vi "Main.vi"() -> ()   [LabVIEW 2014]
uses:
  MAVLink_example.llb/Heartbeat.ctl
  MAVLink_example.llb/Battery Info.ctl
  MAVLink_example.llb/Raw IMU.ctl
  MAVLink_example.llb/Position.ctl
  MAVLink_example.llb/Attitude.ctl
  <vilib>/myRIO/Common/Instrument Driver Framework/myRIO v1.0/PWM/vis/myRIO v1.1 Open PWM.vi
  <vilib>/myRIO/Common/Instrument Driver Framework/myRIO v1.0/UART/vis/myRIO v1.0 Close UART.vi
  <vilib>/myRIO/Common/Instrument Driver Framework/Utilities/vis/Validate Channels.vi
  <vilib>/myRIO/Common/Instrument Driver Framework/myRIO v1.0/PWM/vis/myRIO v1.0 Reserve PWM.vi
  <vilib>/myRIO/Common/Instrument Driver Framework/myRIO v1.0/PWM/vis/myRIO v1.0 Build MUX Configuration PWM.vi
  <vilib>/myRIO/Common/Instrument Driver Framework/myRIO v1.0/Resource Manager/vis/myRIO v1.0 Reserve Channel List.vi
  <vilib>/myRIO/Common/Instrument Driver Framework/myRIO v1.0/Resource Manager/vis/myRIO v1.0 Create Configuration List.vi
  <vilib>/myRIO/Common/Instrument Driver Framework/myRIO v1.0/Resource Manager/vis/myRIO v1.0 Reserve Channel.vi
  <vilib>/myRIO/Common/Instrument Driver Framework/myRIO v1.0/Resource Manager/vis/myRIO v1.0 Unreserve Channel.vi
  <vilib>/myRIO/Common/Instrument Driver Framework/myRIO v1.0/Resource Manager/vis/myRIO v1.0 Build Mutex Name.vi
  <vilib>/Utility/VariantDataType/GetNumericInfo.vi
  <vilib>/Utility/error.llb/Error Cluster From Error Code.vi
  <vilib>/myRIO/Common/Instrument Driver Framework/myRIO v1.0/myRIO v1.1 Open.vi
  <vilib>/myRIO/Common/Instrument Driver Framework/Utilities/vis/IO Manager.vi
  <vilib>/myRIO/Common/Instrument Driver Framework/Utilities/vis/Configuration Manager.vi
  <vilib>/myRIO/Common/Instrument Driver Framework/myRIO v1.0/Resource Manager/vis/myRIO v1.0 Configure IO.vi
  <vilib>/myRIO/Common/Instrument Driver Framework/myRIO v1.0/myRIO v1.0 Close.vi
  Web/Globals/globalAntena.vi
  <vilib>/myRIO/Common/Instrument Driver Framework/myRIO v1.0/PWM/vis/myRIO v1.0 Write PWM.vi
  MAVLink_example.llb/Global Vars.vi
  <vilib>/myRIO/Common/Instrument Driver Framework/Utilities/vis/FPGA Ref Manager.vi
  <vilib>/myRIO/Common/Instrument Driver Framework/myRIO v1.0/myRIO v1.0 Reset FPGA.vi
  <vilib>/myRIO/Common/Instrument Driver Framework/myRIO v1.0/IRQ/vis/myRIO v1.0 IRQ Info FGV.vi
  <vilib>/myRIO/Common/Instrument Driver Framework/myRIO v1.0/IRQ/vis/myRIO v1.0 Timer IRQ Info FGV.vi
  <vilib>/myRIO/Common/Instrument Driver Framework/myRIO v1.0/IRQ/vis/myRIO v1.0 ISR Agent.vi
  Web/Globals/globalAvion.vi
  <vilib>/myRIO/Instrument Drivers/Utilities/Utilities.lvlib
  <vilib>/myRIO/Instrument Drivers/Onboard IO/PWM/PWM.lvlib
panel:
  out "error out 2":errorcluster
  out "Attitude":T1
  out "Position":T2 {"Heading" format="%.2f"}
  out "Raw IMU":T3
  out "Battery Info":T4 {"Batt Voltage (V)" format="%.2f"; "Batt Current (Ah)" format="%.2f"}
  out "HeartBeat":T5 {"custom_mode" format="%x"}
  out "GPS Lock":bool
  out "Received Messages":u8[](array[numeric])
  out "# of HB":u32
  in  "stop":bool
  out "error out":errorcluster
  in  "Actualizar":bool
  out "Altitud Global":dbl
  out "Longitud Global":dbl
  out "Latitud Global":dbl
  in  "Altitud":dbl
  in  "Longitud":dbl
  in  "Latitud":dbl
  in  "Arriba":bool
  in  "Derecha":bool
  out "Duty Cycle  [E]":dbl(graph)
  out "Grados [E]":dbl(graph)
  out "offset [%FS] [E]":dbl
  out "duty cycle [%]  [E]":dbl
  out "pulse width [ms]  [E]":dbl=1.5
  in  "null offset 3":bool
  in  "freq [Hz] Elevación":dbl=50.0
  in  "Parar elevacion":bool
  in  "Kp elevación":dbl=0.05
  in  "Kp rotación":dbl=0.02
  out "Objeto detectado":bool
  in  "Parar rotacion":bool
  out "Grados  [R]":dbl(graph)
  out "Duty Cycle  [R]":dbl(graph)
  out "offset [%FS]  [R]":dbl
  in  "null offset 2":bool
  out "duty cycle [%]  [R]":dbl
  out "pulse width [ms]  [R]":dbl=1.5
  in  "freq [Hz] Rotación":dbl=50.0
  in  "milliseconds to wait":u32=200
  out "Frame Rate":dbl
  in  "Number of Erosion (Adv. Morphology 1)":i32=5
  out "Imagen procesada":T6(plugin-control)
  out "Centroid (Centroid 1)":cluster{"X Centroid":sgl, "Y Centroid":sgl} {"Y Centroid" format="%.2f"; "X Centroid" format="%.2f"}
  out "Number of Particles (Particle Analysis 1)":i32
  in  "Range (Threshold 1)":cluster{"Lower value":sgl, "Upper value":sgl}={"Lower value"=203.0, "Upper value"=255.0}
  in  "Stop (F)":bool
  # "PROCESADO IMAGEN"
  # "DIRECCION RASTREO ->"
  # "ROTACIÓN"
  # "ELEVACIÓN"
  # "POSICION ANTENA"
  # "GPS"
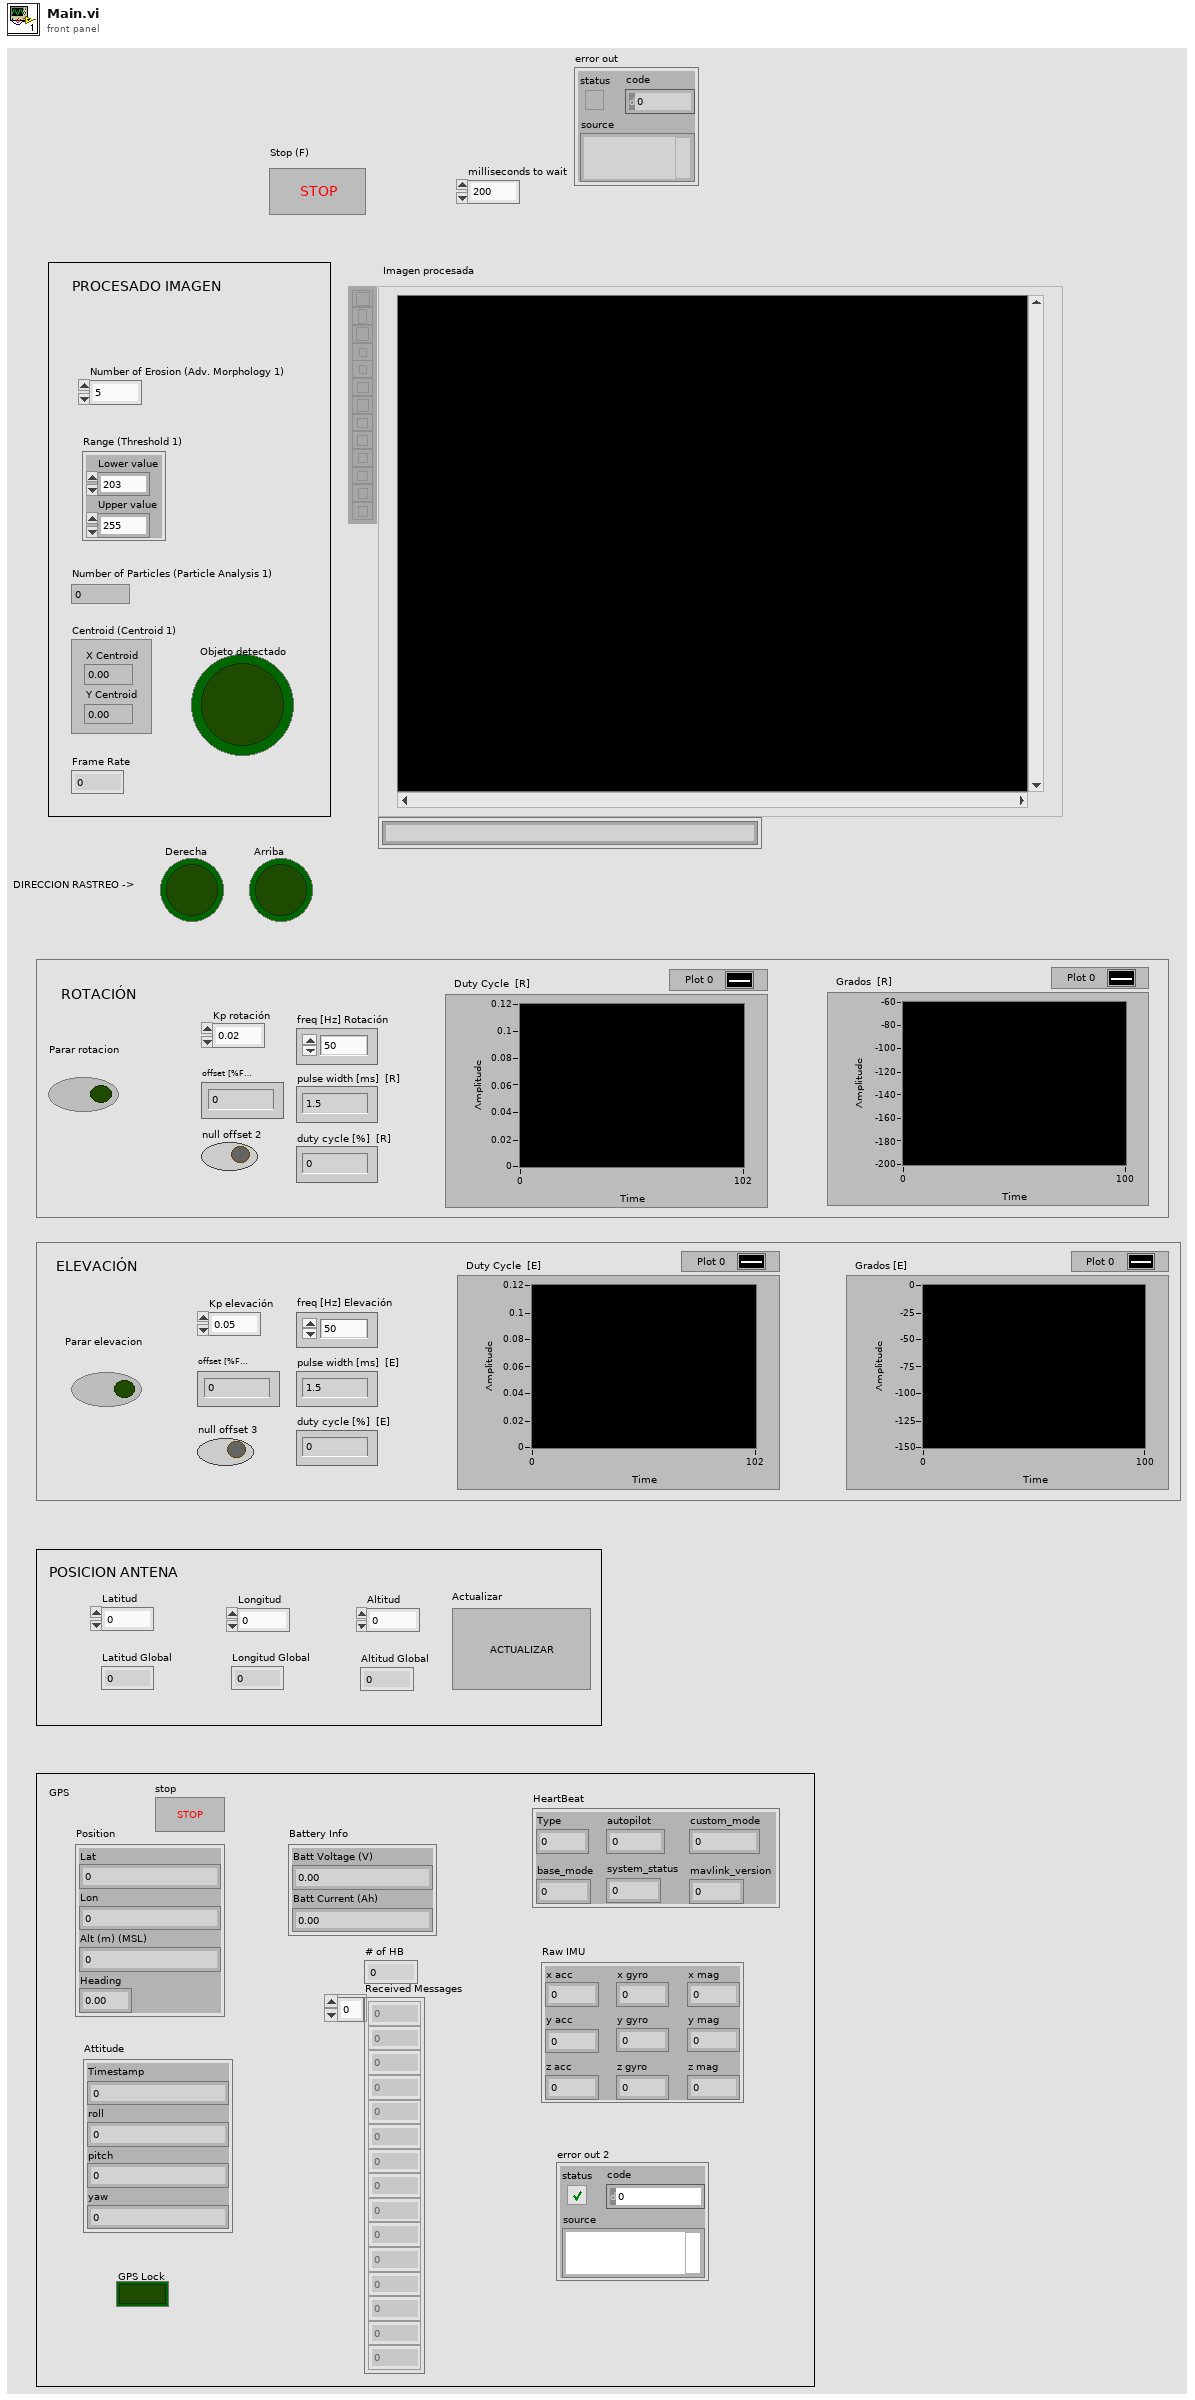
[diagram p1: front panel]
types:
  T1 = typedef "Attitude.ctl" = cluster{"Timestamp":u32, "roll":sgl, "pitch":sgl, "yaw":sgl}
  T2 = typedef "Position.ctl" = cluster{"Lat":sgl, "Lon":sgl, "Alt (m) (MSL)":sgl, "Heading":dbl}
  T3 = typedef "Raw IMU.ctl" = cluster{"x acc":i16, "y acc":i16, "z acc":i16, "x gyro":i16, "y gyro":i16, "z gyro":i16, "x mag":i16, "y mag":i16, "z mag":i16}
  T4 = typedef "Battery Info.ctl" = cluster{"Batt Voltage (V)":dbl, "Batt Current (Ah)":dbl}
  T5 = typedef "Heartbeat.ctl" = cluster{"custom_mode":u32, "Type":u8, "autopilot":u8, "base_mode":u8, "system_status":u8, "mavlink_version":u8}
  T6 = typedef "IMAQ Image.ctl" = refnum<image>
  T7 = typedef "PWM.lvlib/PWM Reference.ctl" = cluster{"myRIO Reference":T8, "PWM Channels Enum":T12, "PWM Configuration":T13}
  T8 = typedef "myRIO Generic Hardware Reference.ctl" = cluster{"myRIO Model":T9, "myRIO Hardware Reference":T10}
  T9 = typedef "Hardware Version Enum.ctl" = enum16{"Unknown", "myRIO-1900", "myRIO-1950"}
  T10 = typedef "myRIO v1.0 Reference.ctl" = cluster{"Generic FPGA Reference":T11, "Allow multiple opens":bool}
  T11 = typedef "Generic FPGA Reference.ctl" = refnum<k20>
  T12 = typedef "PWM Channels Enum.ctl" = enum16{"Not Connected", "C/PWM0", "C/PWM1", "A/PWM0", "A/PWM1", "A/PWM2", "B/PWM0", "B/PWM1", "B/PWM2"}
  T13 = typedef "PWM.lvlib/PWM Configuration.ctl" = cluster{"Frequency":dbl, "Duty Cycle":dbl}
  T14 = typedef "heartbeat.ctl" = cluster{"custom_mode":u32, "Type":u8, "autopilot":u8, "base_mode":u8, "system_status":u8, "mavlink_version":u8}
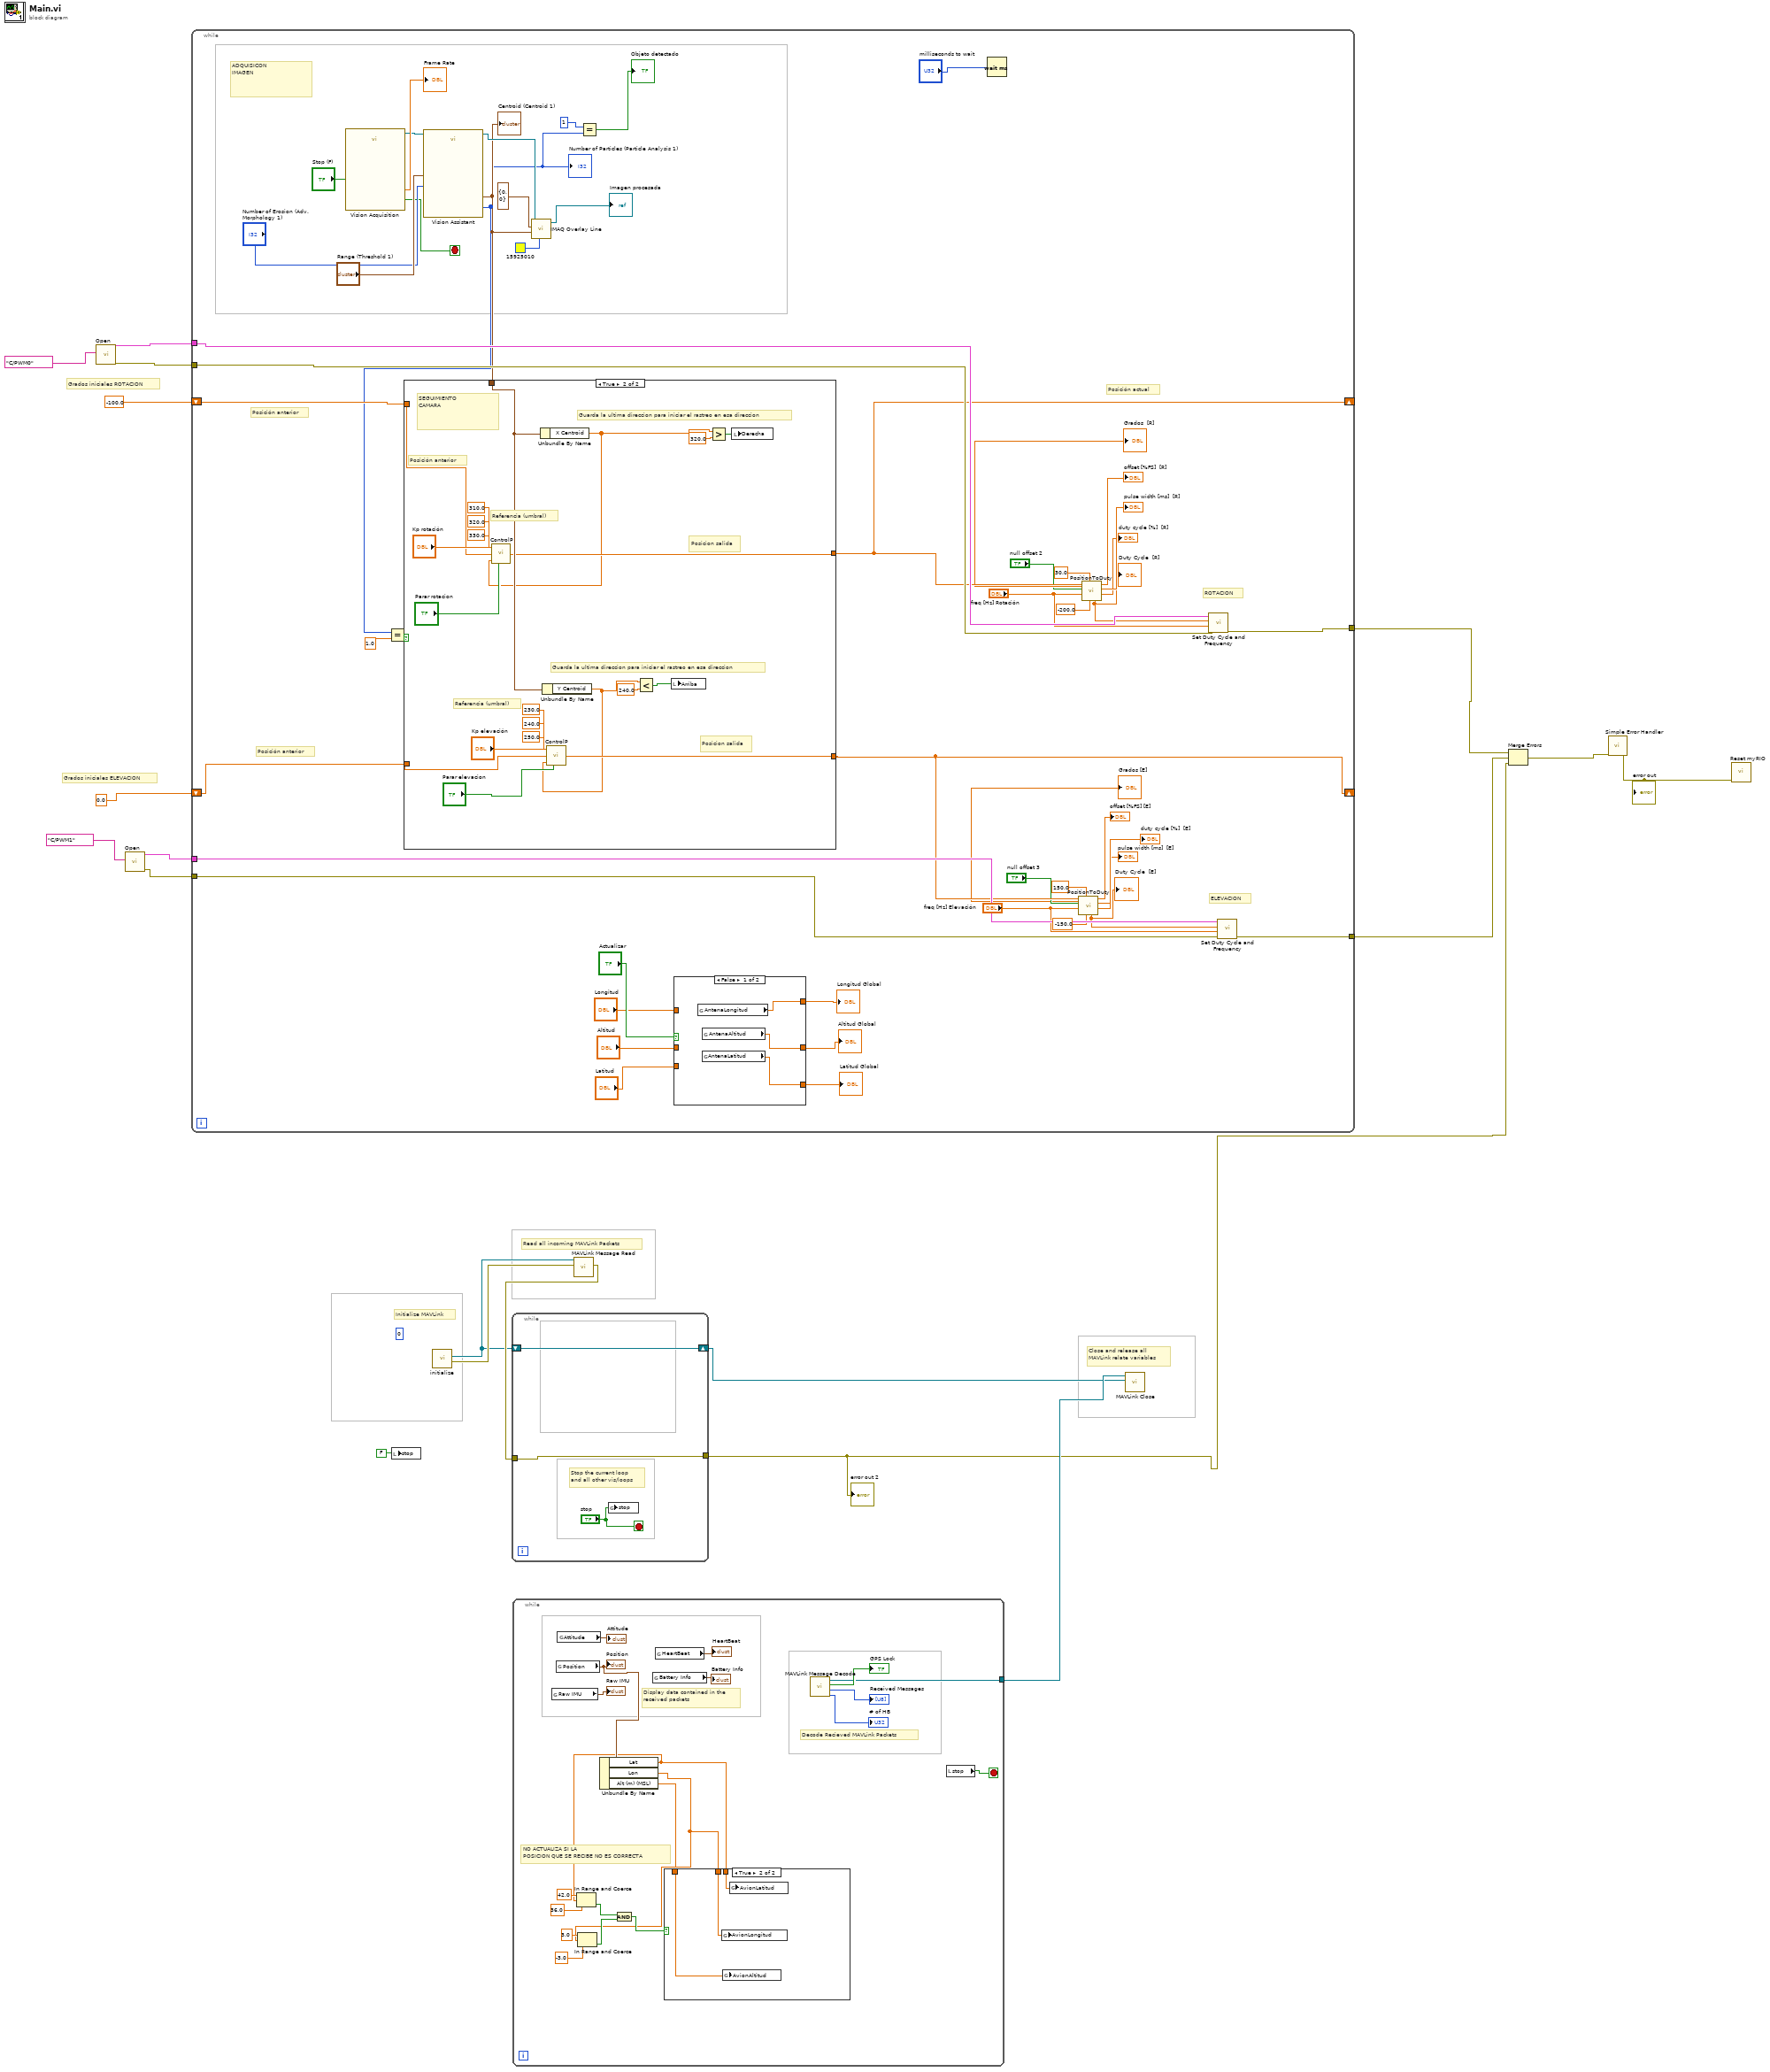
[diagram p0: block diagram]
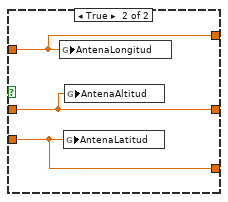
[diagram p3: hidden frame]
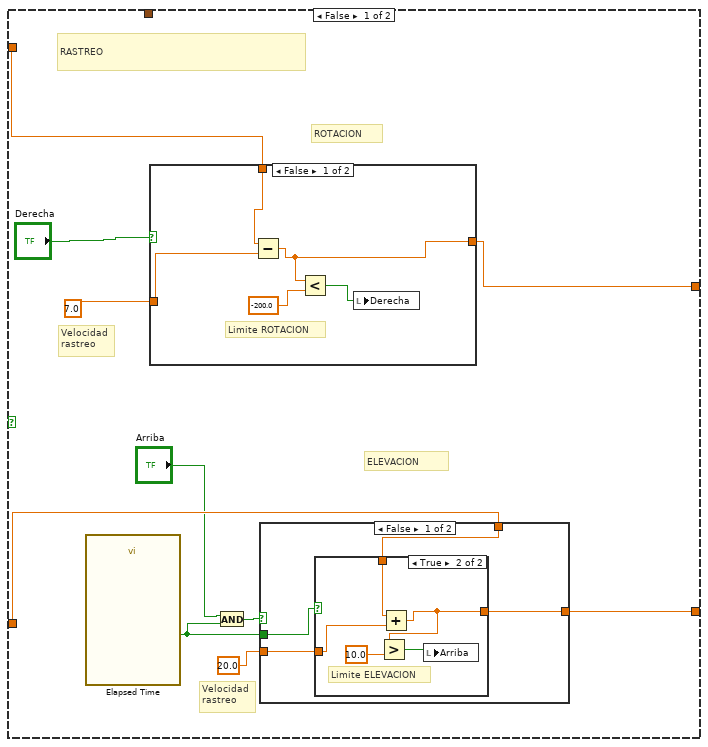
[diagram p4: hidden frame]
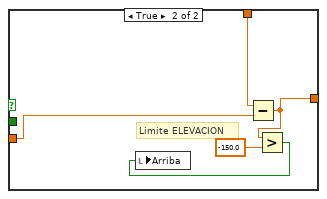
[diagram p6: hidden frame]
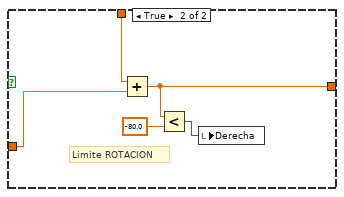
[diagram p7: hidden frame]
diagram:
  (unwired) u8 0 ("Packet Sequence In")
  # "Close and release all\nMAVLink relate variables"
  # "Read all incoming MAVLink Packets"
  # "Initialize MAVLink"
  # "Grados iniciales ELEVACION"
  # "Grados iniciales ROTACION"
  n1 = call <vilib>:"Open.vi"("Channel Name"=tag "C/PWM0" ("PWM channel")) -> ("error out"=w16:errorcluster, "PWM Ref Out"=w17:T7)  [unwired: 9 in]
  n2 = call <vilib>:"Open.vi"("Channel Name"=tag "C/PWM1" ("PWM channel")) -> ("error out"=w12:errorcluster, "PWM Ref Out"=w13:T7)  [unwired: 9 in]
  n3 = while {
    tunnel: w17 -> [w61]
    tunnel: w16 -> [w60]
    tunnel: [w51] -> w11
    shift-right: [w47] -> _
    shift-left: -100.0 -> [w53]
    tunnel: w13 -> [w56]
    tunnel: w12 -> [w55]
    shift-right: [w36] -> _
    shift-left: 0.0 -> [w52]
    tunnel: [w50] -> w8
    stop <- w63 stop-if-true
    # "ADQUISICON\nIMAGEN"
    # "Posición anterior"
    # "ELEVACION"
    # "ROTACION"
    # "Posición actual"
    # "Posición anterior"
    n4 = call "Vision Acquisition"("Stop (F)"="Stop (F)") -> ("Image Out"=w65:T6, "Frame Rate"=→"Frame Rate":dbl, "Stopped"=w63:bool)  [unwired: 23 in, 1 out]
    n5 = call "Vision Assistant"("Image In"=w65, "Range (Threshold 1)"="Range (Threshold 1)", "Number of Erosion (Adv. Morphology 1)"="Number of Erosion (Adv. Morphology 1)") -> ("Image Out"=w68:T6, "Centroid (Centroid 1)"=w54:cluster{"X Centroid":sgl, "Y Centroid":sgl}, "Number of Particles (Particle Analysis 1)"=w48:i32)  [unwired: 21 in, 1 out]
    "Number of Particles (Particle Analysis 1)" <- w48
    "Centroid (Centroid 1)" <- w54
    n6 = Equal?(x=w48, y=1.0) -> (x = y?=w27:bool)
    n7 = case shown="True" w27 {
      tunnel: w54 -> [_ w133]
      tunnel: w53 -> [w87 w131]
      tunnel: [w79 w130] -> w47
      tunnel: w52 -> [w84 w124]
      tunnel: [w78 w122] -> w36
      frame False {
        # "ROTACION"
        # "ELEVACION"
        # "Velocidad\nrastreo"
        # "Velocidad\nrastreo"
        # "RASTREO"
        n8 = call "Elapsed Time"() -> ("Time has Elapsed"=w81:bool)  [unwired: 12 in, 7 out]
        n9 = case shown="False" "Derecha" {
          tunnel: w87 -> [w106 w112]
          tunnel: [w105 w110] -> w79
          tunnel: 7.0 ("y") -> [w104 w108]
          frame False {
            # "Limite ROTACION"
            n10 = Subtract(x=w106, y=w104) -> (x-y=w105:dbl)
            n11 = Less?(x=w105, y=-200.0) -> (x < y?=w103:bool)
            n12 = local write "Derecha"(w103) -> ()
          }
          frame True {
            # "Limite ROTACION"
            n13 = Add(x=w112, y=w108) -> (x+y=w110:dbl)
            n14 = Less?(x=w110, y=-80.0) -> (x < y?=w109:bool)
            n15 = local write "Derecha"(w109) -> ()
          }
        }
        n16 = And(x="Arriba", y=w81) -> (x .and. y?=w82:bool)
        n17 = case shown="False" w82 {
          tunnel: w84 -> [w90 w102]
          tunnel: [w89 w101] -> w78
          tunnel: w81 -> [w91 _]
          tunnel: 20.0 ("y") -> [w88 w98]
          frame False {
            n18 = case shown="True" w91 {
              tunnel: w90 -> [w92 w97]
              tunnel: [w92 w96] -> w89
              tunnel: w88 -> [_ w93]
              frame False {
              }
              frame True {
                # "Limite ELEVACION"
                n19 = Add(x=w97, y=w93) -> (x+y=w96:dbl)
                n20 = Greater?(x=w96, y=10.0) -> (0:w94:bool)
                n21 = local write "Arriba"(w94) -> ()
              }
            }
          }
          frame True {
            # "Limite ELEVACION"
            n22 = Subtract(x=w102, y=w98) -> (x-y=w101:dbl)
            n23 = Greater?(x=w101, y=-150.0) -> (0:w99:bool)
            n24 = local write "Arriba"(w99) -> ()
          }
        }
      }
      frame True {
        # "Posicion salida"
        # "Posición anterior"
        # "Referencia (umbral)"
        # "Referencia (umbral)"
        # "SEGUIMIENTO\nCAMARA"
        # "Guarda la ultima direccion para iniciar el rastreo en esa direccion"
        # "Guarda la ultima direccion para iniciar el rastreo en esa direccion"
        # "Posicion salida"
        n25 = Unbundle By Name(w133) -> ("X Centroid"=w114:sgl)
        n26 = call "ControlP.vi"("Kp"="Kp rotación", "Referencia superior"=330.0, "Posición anterior"=w131, "Coordenada X o Y"=w114, "Parar"="Parar rotacion", "Referencia"=320.0, "Referencia inferior"=310.0) -> ("Posición"=w130:dbl)  [unwired: 2 in]
        n27 = Unbundle By Name(w133) -> ("Y Centroid"=w113:sgl)
        n28 = call "ControlP.vi"("Kp"="Kp elevación", "Referencia superior"=250.0, "Posición anterior"=w124, "Coordenada X o Y"=w113, "Parar"="Parar elevacion", "Referencia"=240.0, "Referencia inferior"=230.0) -> ("Posición"=w122:dbl)  [unwired: 2 in]
        n29 = Less?(x=w113, y=sgl 240.0) -> (x < y?=w115:bool)
        n30 = local write "Arriba"(w115) -> ()
        n31 = Greater?(x=w114, y=sgl 320.0) -> (0:w117:bool)
        n32 = local write "Derecha"(w117) -> ()
      }
    }
    n33 = call "IMAQ Overlay Line"("Color"=u32 15925010, "End Point"=w54, "Start Point"=cluster{"X":i32, "Y":i32} {"X"=0, "Y"=0}, "Image"=w68) -> ("Image Out"=→"Imagen procesada":T6)  [unwired: 6 in, 1 out]
    n34 = Equal?(x=1, y=w48) -> (x = y?=→"Objeto detectado":bool)
    n35 = case shown="False" "Actualizar" {
      tunnel: "Longitud" -> [_ w77]
      tunnel: "Altitud" -> [_ w76]
      tunnel: "Latitud" -> [_ w75]
      tunnel: [w74 w77] -> w22
      tunnel: [w73 w76] -> w21
      tunnel: [w72 w75] -> w20
      frame False {
        n36 = global read "globalAntena.vi" "AntenaLongitud"() -> (w74:dbl)
        n37 = global read "globalAntena.vi" "AntenaLatitud"() -> (w72:dbl)
        n38 = global read "globalAntena.vi" "AntenaAltitud"() -> (w73:dbl)
      }
      frame True {
        n39 = global write "globalAntena.vi" "AntenaLongitud"(w77) -> ()
        n40 = global write "globalAntena.vi" "AntenaLatitud"(w75) -> ()
        n41 = global write "globalAntena.vi" "AntenaAltitud"(w76) -> ()
      }
    }
    "Altitud Global" <- w21
    "Longitud Global" <- w22
    "Latitud Global" <- w20
    n42 = Wait (ms)(milliseconds to wait="milliseconds to wait") -> ()  [unwired: 1 out]
    n43 = call "PositionToDuty.vi"("lower limit"=-150.0, "upper limit"=150.0, "freq [Hz] in"="freq [Hz] Elevación", "null offset in"="null offset 3", "Posición"=w36) -> ("duty cycle [%] 2"=→"duty cycle [%]  [E]":dbl, "pulse width [ms] 2"=→"pulse width [ms]  [E]":dbl, "offset [%FS] 2"=→"offset [%FS] [E]":dbl, "DutyCycle"=w28:dbl, "Grados"=→"Grados [E]":dbl)  [unwired: 2 in]
    "Duty Cycle  [E]" <- w28
    n44 = call "PositionToDuty.vi"("lower limit"=-200.0, "upper limit"=30.0, "freq [Hz] in"="freq [Hz] Rotación", "null offset in"="null offset 2", "Posición"=w47) -> ("duty cycle [%] 2"=→"duty cycle [%]  [R]":dbl, "pulse width [ms] 2"=→"pulse width [ms]  [R]":dbl, "offset [%FS] 2"=→"offset [%FS]  [R]":dbl, "DutyCycle"=w40:dbl, "Grados"=→"Grados  [R]":dbl)  [unwired: 2 in]
    "Duty Cycle  [R]" <- w40
    n45 = call <vilib>:"Set Duty Cycle and Frequency.vi"("error in (no error)"=w60, "Frequency [Hz]"="freq [Hz] Rotación", "Duty Cycle"=w40, "PWM Ref In"=w61) -> ("error out"=w51:errorcluster)  [unwired: 5 in, 1 out]
    n46 = call <vilib>:"Set Duty Cycle and Frequency.vi"("error in (no error)"=w55, "Frequency [Hz]"="freq [Hz] Elevación", "Duty Cycle"=w28, "PWM Ref In"=w56) -> ("error out"=w50:errorcluster)  [unwired: 5 in, 1 out]
  }
  n47 = local write "stop"(FALSE ("stop")) -> ()
  n48 = call "initialize.vi"() -> ("error out"=w4:errorcluster, "VISA resource name"=w3:refnum<visa-resource-name>)  [unwired: 10 in]
  n49 = while {
    tunnel: [w146] -> w7
    stop <- w145 stop-if-true
    # "NO ACTUALIZA SI LA\nPOSICION QUE SE RECIBE NO ES CORRECTA"
    # "Decode Recieved MAVLink Packets"
    # "Display data contained in the\nreceived packets"
    n50 = global read "Global Vars.vi" "Raw IMU"() -> (→"Raw IMU":T3)
    n51 = global read "Global Vars.vi" "Position"() -> (w144:T2)
    "Position" <- w144
    n52 = global read "Global Vars.vi" "Attitude"() -> (→"Attitude":T1)
    n53 = Unbundle By Name(w144) -> ("Lat"=w136:sgl, "Lon"=w135:sgl, "Alt (m) (MSL)"=w134:sgl)
    n54 = In Range and Coerce(upper limit=42.0, x=w136, lower limit=36.0) -> (In Range?=w139:bool)  [unwired: 1 out]
    n55 = In Range and Coerce(upper limit=3.0, x=w135, lower limit=-3.0) -> (In Range?=w138:bool)  [unwired: 1 out]
    n56 = And(x=w139, y=w138) -> (x .and. y?=w137:bool)
    n57 = global read "Global Vars.vi" "Battery Info"() -> (→"Battery Info":T4)
    n58 = global read "Global Vars.vi" "HeartBeat"() -> (→"HeartBeat":T14)
    n59 = case shown="True" w137 {
      tunnel: w136 -> [_ w156]
      tunnel: w135 -> [_ w155]
      tunnel: w134 -> [_ w154]
      frame False {
      }
      frame True {
        n60 = global write "globalAvion.vi" "AvionLongitud"(w155) -> ()
        n61 = global write "globalAvion.vi" "AvionAltitud"(w154) -> ()
        n62 = global write "globalAvion.vi" "AvionLatitud"(w156) -> ()
      }
    }
    n63 = call "MAVLink Message Decode.vi"() -> ("# of HB"=→"# of HB":u32, "Received Messages"=→"Received Messages":u8[], "GPS Lock"=→"GPS Lock":bool, "queue out"=w146:refnum<queue>)  [unwired: 8 in]
    n64 = local read "stop"() -> (w145:bool)
  }
  n65 = call "MAVLink Message Read.vi"("error out 2"=w4, "MAVLink Com Port IN"=w3) -> ("error out"=w5:errorcluster)  [unwired: 8 in, 1 out]
  n66 = while {
    shift-right: [w158] -> w2
    shift-left: w3 -> [w158]
    tunnel: w5 -> [w157]
    tunnel: [w157] -> w1
    stop <- "stop" stop-if-true
    # "Stop the current loop\nand all other vis/loops"
    n67 = global write "Global Vars.vi" "stop"("stop") -> ()
  }
  "error out 2" <- w1
  n68 = call "MAVLink Close.vi"("MAVLink Com Port In"=w2, "queue"=w7) -> ()  [unwired: 10 in]
  n69 = Merge Errors(w11, w8, w1) -> (w10:errorcluster)
  n70 = call <vilib>:"Simple Error Handler.vi"("error in (no error)"=w10) -> ("error out"=w18:errorcluster)  [unwired: 4 in, 4 out]
  "error out" <- w18
  n71 = call <vilib>:"Reset myRIO.vi"("error in (no error)"=w18) -> ()  [unwired: 10 in, 1 out]
